vi "ReadAndProcessCommand.vi"(11 "MockGyroData In":T1={"BufferUpdateFIFO"="MockGyroBufferUpdate", "MockGyroCommandInput"="ModbusSubnetEGyroRxDataFIFO", "MockGyroDataOutput"="ModbusSubnetEGyroTxDataFIFO", "MockGyroDataRate"="MockGyroDataRateRegister", "MockGyroXValue"="MockGyroXValueRegister", "MockGyroYValue"="MockGyroYValueRegister", "MockGyroZValue"="MockGyroZValueRegister", "MockGyroStatus"="MockGyroStatusRegister", "MockGyroTemperature"="MockGyroTemperatureRegister", "CRCDataFIFO"="MockGyroCRCDataFIFO", "CRCCalculateFIFO"="MockGyroCRCCalculateFIFO", "CRCFIFO"="MockGyroCRCFIFO", "MockGyroCommandReplyFIFO"="MockGyroCommandReplyFIFO", "MockGyroReplyReadyFIFO"="MockGyroReplyReadyFIFO", "MockGyroModeFIFO"="MockGyroModeFIFO"}) -> ()   [LabVIEW 2016, in "FPGAMockGyro.lvlib"]
uses:
  FPGAMockGyro.lvlib
  DataTypes/MockGyroData.ctl
  DataTypes/MockGyroModes.ctl
  <vilib>/rvi/Emulation/niFpgaGetClockAttributes.vi
  <vilib>/rvi/Emulation/niFpgaSctlEmulationGetInTimedLoop.vi
  <vilib>/rvi/Emulation/niFpgaEmulationReportErrorSimple.vi
  <vilib>/rvi/DataTransferAndStorage/Container/Common/niFpgaContainerExecOnDevCompGetState.vi
  <vilib>/rvi/Emulation/niFpgaEmulationIsFPGAContextNoSignature.vi
  <vilib>/rvi/errors/niFpgaSetErrorForExecOnDevCompSimple.vi
  <vilib>/rvi/eio/common/nirviEmuReportErrorAndStop.vi
  <vilib>/rvi/DataTransferAndStorage/Container/Common/niFpgaContainerGetUniqueNameForEmu.vi
  <vilib>/rvi/FIFO/Fifo_Resource/nirvififoEmulationSetSize.vi
  <vilib>/rvi/FIFO/Fifo_Resource/nirviFifoEmulationQueueMgr.vi
  <instcachedir>/0/nirviFifoEmulationQueueMgr_E5CAEC123FF24DC58D834DCA3CDAA9B5.lvgen/nirviFifoEmulationQueueMgr_E5CAEC123FF24DC58D834DCA3CDAA9B5_002.vi
  <vilib>/rvi/FIFO/Fifo_Resource/nirvififoEmulationDetermineInputValidOut.vi
  <vilib>/rvi/FIFO/Fifo_Resource/nirvififoEmulationCreateLock.vi
  <vilib>/rvi/Emulation/niFpgaProcessEmulError.vi
  <vilib>/rvi/FIFO/Fifo_Resource/nirvififoEmulationObtainLock.vi
  <vilib>/rvi/FIFO/Fifo_Resource/nirvififoEmulationReleaseLock.vi
  <vilib>/rvi/occurrence/nirviWaitOnOccurrenceBase.vi
  <vilib>/rvi/errors/nirviReportUnexpectedCaseInternalError.vi
  <vilib>/rvi/errors/nirviReportUnexpectedCaseInternalError (U32).vi
  <vilib>/Utility/error.llb/Clear Errors.vi
  <vilib>/rvi/interface/RandomDataEmulation/niFpgaRandomDataHandleErrors.vi
  <instcachedir>/0/nirviFifoEmulationQueueMgr_E5CAEC123FF24DC58D834DCA3CDAA9B5.lvgen/nirviFifoEmulationQueueMgr_E5CAEC123FF24DC58D834DCA3CDAA9B5_000.vi
  <vilib>/rvi/Emulation/niFpgaCriticalErrorInLSC.vi
  <vilib>/rvi/Memory/Memory_Emulation/niFpgaMemoryEmulationCacheClearOnFirstRun.vi
  <vilib>/rvi/Memory/Memory_Emulation/nirvimemoryEmulationManagerCache_MakeExclusive.vi
  <vilib>/rvi/Memory/Memory_Emulation/niFpgaMemoryEmulationValidateCache.vi
  <vilib>/rvi/Memory/Memory_Emulation/nirvimemoryEmulationManagerCache_InsertValue.vi
  <vilib>/rvi/Memory/Memory_Emulation/nirvimemoryEmulationManagerCache_ReleaseExclusive.vi
  <vilib>/rvi/Memory/Memory_Emulation/nirvimemoryEmulationManagerCache_GetValue.vi
  <vilib>/rvi/Memory/Memory_Emulation/nirvimemoryEmulationManagerCache_SetValue.vi
  <instcachedir>/0/nirviFifoEmulationQueueMgr_E5CAEC123FF24DC58D834DCA3CDAA9B5.lvgen/nirviFifoEmulationQueueMgr_E5CAEC123FF24DC58D834DCA3CDAA9B5_001.vi
  <vilib>/rvi/DataTransferAndStorage/Container/XNode/niFpgaContainer.xnode
  <vilib>/rvi/FIFO/Fifo_Resource/niFpgaFifoEmulationRefIn.vi
  <vilib>/rvi/DataTransferAndStorage/Register/Emulation/niFpgaRegisterEmulationRefIn.vi
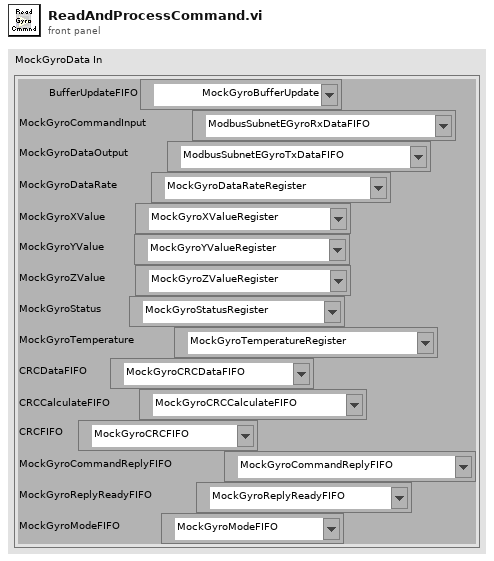
[diagram p1: front panel]
types:
  T1 = typedef "FPGAMockGyro.lvlib/MockGyroData.ctl" = cluster{"BufferUpdateFIFO":refnum<k21>, "MockGyroCommandInput":refnum<k21>, "MockGyroDataOutput":refnum<k21>, "MockGyroDataRate":refnum<k21>, "MockGyroXValue":refnum<k21>, "MockGyroYValue":refnum<k21>, "MockGyroZValue":refnum<k21>, "MockGyroStatus":refnum<k21>, "MockGyroTemperature":refnum<k21>, "CRCDataFIFO":refnum<k21>, "CRCCalculateFIFO":refnum<k21>, "CRCFIFO":refnum<k21>, "MockGyroCommandReplyFIFO":refnum<k21>, "MockGyroReplyReadyFIFO":refnum<k21>, "MockGyroModeFIFO":refnum<k21>}
  T2 = typedef "FPGAMockGyro.lvlib/MockGyroModes.ctl" = enum8{"Normal", "Config"}
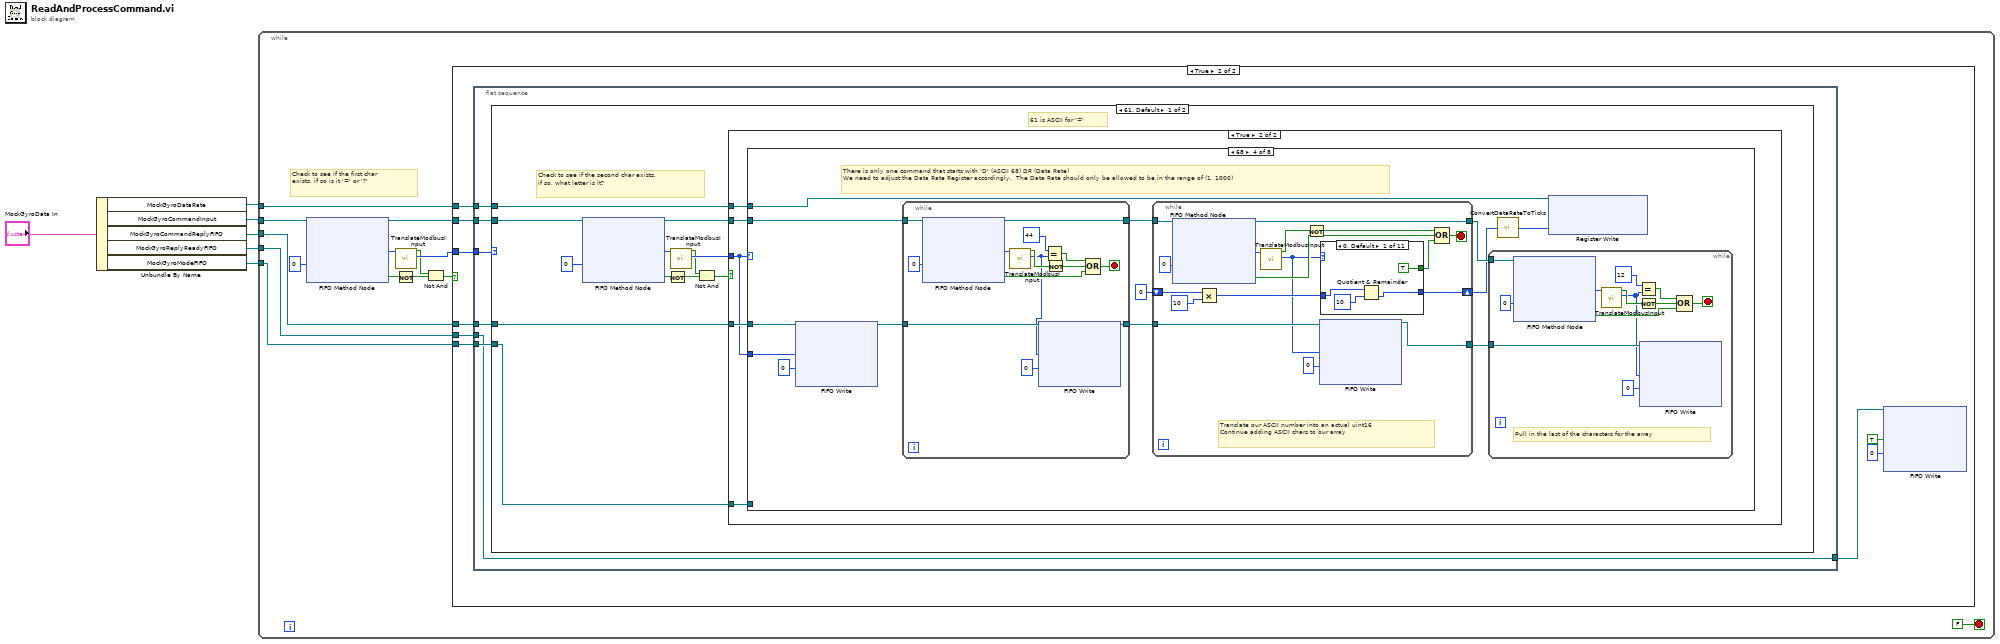
[diagram p0: block diagram]
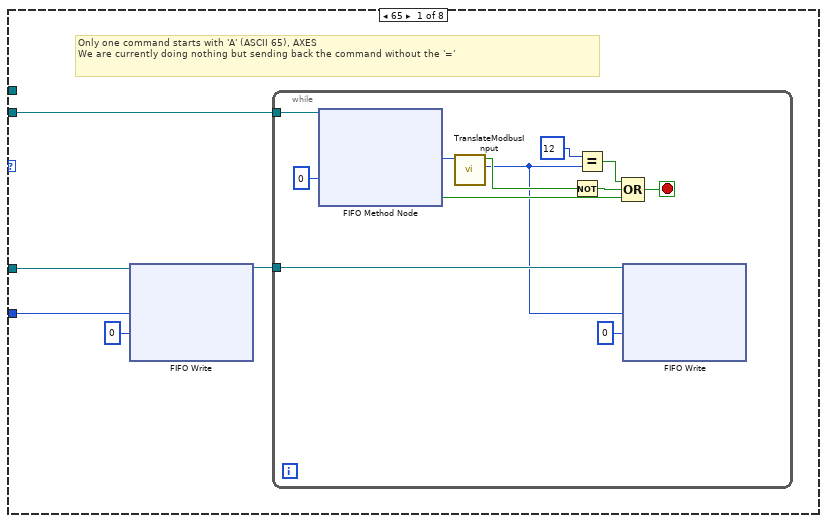
[diagram p4: hidden frame]
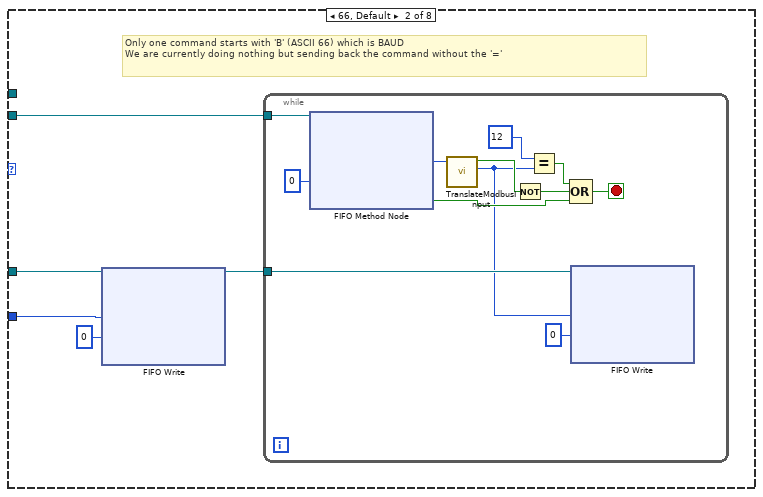
[diagram p5: hidden frame]
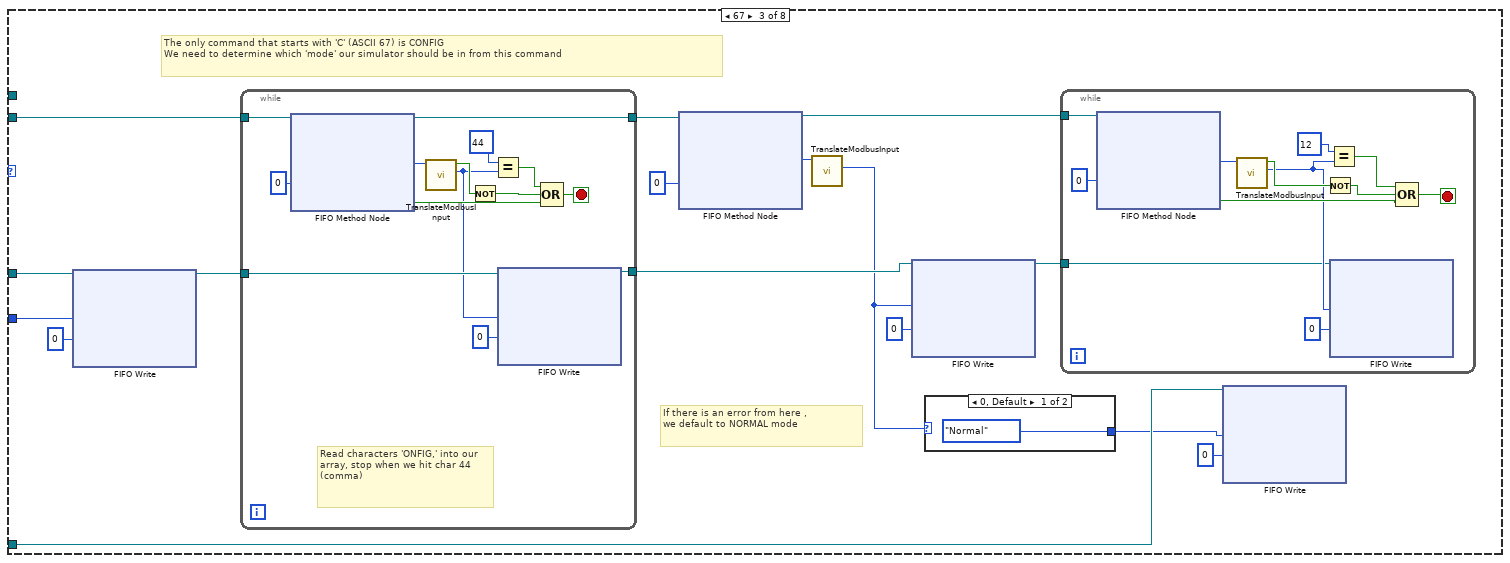
[diagram p6: hidden frame]
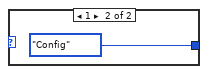
[diagram p7: hidden frame]
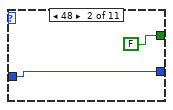
[diagram p8: hidden frame]
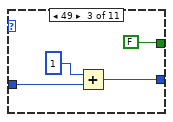
[diagram p9: hidden frame]
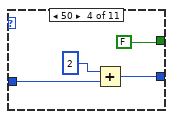
[diagram p10: hidden frame]
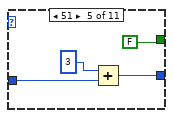
[diagram p11: hidden frame]
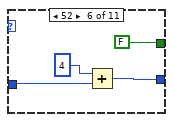
[diagram p12: hidden frame]
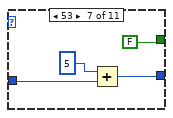
[diagram p13: hidden frame]
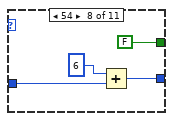
[diagram p14: hidden frame]
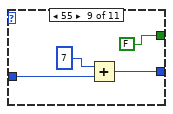
[diagram p15: hidden frame]
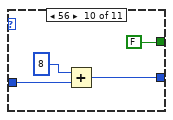
[diagram p16: hidden frame]
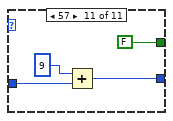
[diagram p17: hidden frame]
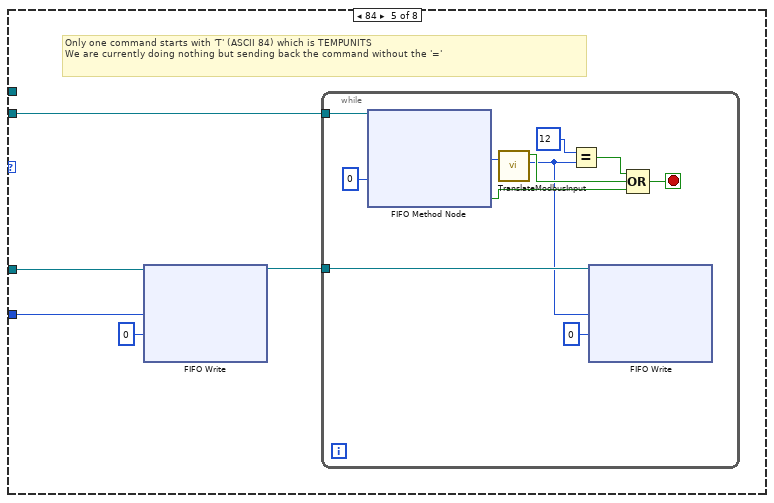
[diagram p18: hidden frame]
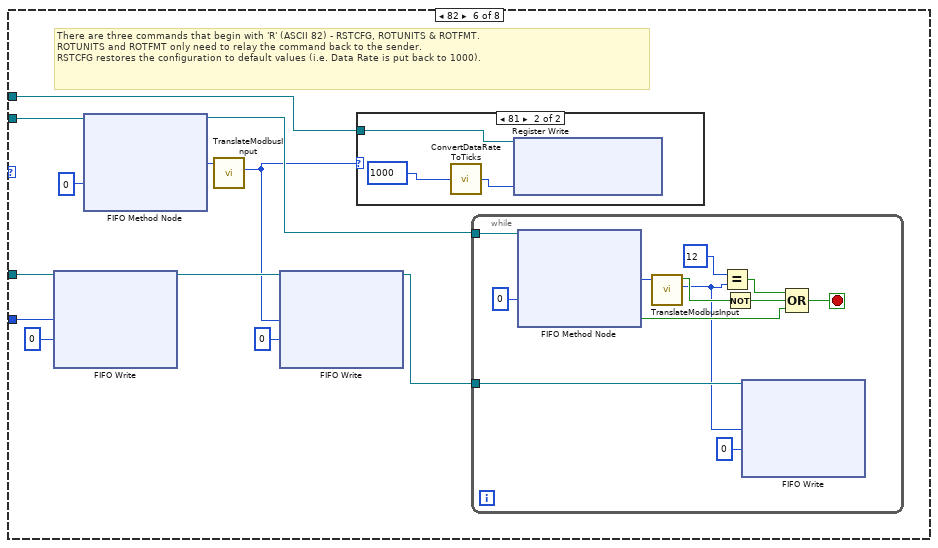
[diagram p19: hidden frame]
diagram:
  n1 = Unbundle By Name("MockGyroData In") -> ("MockGyroDataRate"=w4:refnum<k21>, "MockGyroCommandInput"=w6:refnum<k21>, "MockGyroCommandReplyFIFO"=w3:refnum<k21>, "MockGyroReplyReadyFIFO"=w2:refnum<k21>, "MockGyroModeFIFO"=w1:refnum<k21>)
  n2 = while {
    tunnel: w6 -> [w19]
    tunnel: w4 -> [w17]
    tunnel: w3 -> [w9]
    tunnel: w2 -> [w8]
    tunnel: w1 -> [w7]
    stop <- FALSE stop-if-true
    # "Check to see if the first char \nexists, if so is it '=' or '?'"
    n3 = xnode ("FIFO Method Node")("Timeout"=0, "FIFO In"=w19) -> ("Element"=w16:u16, "Timed Out?"=w14:bool, "FIFO Out"=w18:refnum<k21>)
    n4 = call "TranslateModbusInput.vi"("ModbusInput"=w16) -> ("ASCII Number Output"=w15:u8, "Is Data?"=w12:bool)  [unwired: 9 in]
    n5 = Not(x=w14) -> (.not. x?=w11:bool)
    n6 = Not And(1:w11, 2:w12) -> (0:w13:bool)
    n7 = case shown="True" w13 {
      tunnel: w18 -> [_ w29]
      tunnel: w17 -> [_ w28]
      tunnel: w15 -> [_ w27]
      tunnel: w9 -> [_ w26]
      tunnel: w8 -> [_ w23]
      tunnel: w7 -> [_ w25]
      frame False {
      }
      frame True {
        n8 = flat-sequence {
          tunnel: w29 -> [w35]
          tunnel: w28 -> [w34]
          tunnel: w27 -> [w33]
          tunnel: w26 -> [w32]
          tunnel: w25 -> [w31]
          tunnel: w23 -> [w30]
          tunnel: [w30] -> w22
          frame #0 {
            n9 = case shown="61, Default" w33 {
              tunnel: w35 -> [w47 w325]
              tunnel: w34 -> [w44 _]
              tunnel: w32 -> [w37 w324]
              tunnel: w31 -> [w36 _]
              frame 61, Default {
                # "Check to see if the second char exists,\nif so, what letter is it?"
                # "61 is ASCII for '='"
                n10 = xnode ("FIFO Method Node")("Timeout"=0, "FIFO In"=w47) -> ("Element"=w43:u16, "Timed Out?"=w40:bool, "FIFO Out"=w45:refnum<k21>)
                n11 = Not(x=w40) -> (.not. x?=w41:bool)
                n12 = call "TranslateModbusInput.vi"("ModbusInput"=w43) -> ("ASCII Number Output"=w42:u8, "Is Data?"=w39:bool)  [unwired: 9 in]
                n13 = Not And(1:w41, 2:w39) -> (0:w38:bool)
                n14 = case shown="True" w38 {
                  tunnel: w45 -> [_ w52]
                  tunnel: w44 -> [_ w51]
                  tunnel: w42 -> [_ w49]
                  tunnel: w37 -> [_ w50]
                  tunnel: w36 -> [_ w48]
                  frame False {
                  }
                  frame True {
                    n15 = case shown="68" w49 {
                      tunnel: w52 -> [w57 w74 w101 w143 w233 w256 w276 w293]
                      tunnel: w51 -> [_ _ _ w139 _ w253 _ _]
                      tunnel: w50 -> [w56 w73 w98 w138 w232 w251 w274 w292]
                      tunnel: w49 -> [w55 w72 w97 w137 w231 w249 w273 w291]
                      tunnel: w48 -> [_ _ w89 _ _ _ _ _]
                      frame 65 {
                        # "Only one command starts with 'A' (ASCII 65), AXES\nWe are currently doing nothing but sending back the command without the '='"
                        n16 = xnode ("FIFO Write")("Element"=w55, "Timeout"=0, "FIFO In"=w56) -> ("FIFO Out"=w53:refnum<k21>)  [unwired: 1 out]
                        n17 = while {
                          tunnel: w57 -> [w69]
                          tunnel: w53 -> [w60]
                          stop <- w61 stop-if-true
                          n18 = xnode ("FIFO Method Node")("Timeout"=0, "FIFO In"=w69) -> ("Element"=w67:u16, "Timed Out?"=w62:bool)  [unwired: 1 out]
                          n19 = call "TranslateModbusInput.vi"("ModbusInput"=w67) -> ("ASCII Number Output"=w59:u8, "Is Data?"=w64:bool)  [unwired: 9 in]
                          n20 = Not(x=w64) -> (.not. x?=w63:bool)
                          n21 = Equal?(x=u8 12, y=w59) -> (x = y?=w65:bool)
                          n22 = Compound Arithmetic op=OR(w65, w63, w62) -> (w61:bool)
                          n23 = xnode ("FIFO Write")("Element"=w59, "Timeout"=0, "FIFO In"=w60) -> ()  [unwired: 2 out]
                        }
                      }
                      frame 66, Default {
                        # "Only one command starts with 'B' (ASCII 66) which is BAUD\nWe are currently doing nothing but sending back the command without the '='"
                        n24 = xnode ("FIFO Write")("Element"=w72, "Timeout"=0, "FIFO In"=w73) -> ("FIFO Out"=w70:refnum<k21>)  [unwired: 1 out]
                        n25 = while {
                          tunnel: w74 -> [w86]
                          tunnel: w70 -> [w77]
                          stop <- w78 stop-if-true
                          n26 = xnode ("FIFO Method Node")("Timeout"=0, "FIFO In"=w86) -> ("Element"=w84:u16, "Timed Out?"=w79:bool)  [unwired: 1 out]
                          n27 = call "TranslateModbusInput.vi"("ModbusInput"=w84) -> ("ASCII Number Output"=w76:u8, "Is Data?"=w81:bool)  [unwired: 9 in]
                          n28 = Not(x=w81) -> (.not. x?=w80:bool)
                          n29 = Equal?(x=u8 12, y=w76) -> (x = y?=w82:bool)
                          n30 = Compound Arithmetic op=OR(w82, w80, w79) -> (w78:bool)
                          n31 = xnode ("FIFO Write")("Element"=w76, "Timeout"=0, "FIFO In"=w77) -> ()  [unwired: 2 out]
                        }
                      }
                      frame 67 {
                        # "If there is an error from here ,\nwe default to NORMAL mode"
                        # "The only command that starts with 'C' (ASCII 67) is CONFIG\nWe need to determine which 'mode' our simulator should be in from this command"
                        n32 = xnode ("FIFO Write")("Element"=w97, "Timeout"=0, "FIFO In"=w98) -> ("FIFO Out"=w95:refnum<k21>)  [unwired: 1 out]
                        n33 = while {
                          tunnel: w101 -> [w128]
                          tunnel: [w126] -> w99
                          tunnel: w95 -> [w118]
                          tunnel: [w115] -> w94
                          stop <- w119 stop-if-true
                          # "Read characters 'ONFIG,' into our array, stop when we hit char 44 (comma)"
                          n34 = xnode ("FIFO Method Node")("Timeout"=0, "FIFO In"=w128) -> ("Element"=w125:u16, "Timed Out?"=w120:bool, "FIFO Out"=w126:refnum<k21>)
                          n35 = call "TranslateModbusInput.vi"("ModbusInput"=w125) -> ("ASCII Number Output"=w117:u8, "Is Data?"=w122:bool)  [unwired: 9 in]
                          n36 = Not(x=w122) -> (.not. x?=w121:bool)
                          n37 = Equal?(x=u8 44, y=w117) -> (x = y?=w123:bool)
                          n38 = xnode ("FIFO Write")("Element"=w117, "Timeout"=0, "FIFO In"=w118) -> ("FIFO Out"=w115:refnum<k21>)  [unwired: 1 out]
                          n39 = Compound Arithmetic op=OR(w123, w121, w120) -> (w119:bool)
                        }
                        n40 = xnode ("FIFO Method Node")("Timeout"=0, "FIFO In"=w99) -> ("Element"=w100:u16, "FIFO Out"=w91:refnum<k21>)  [unwired: 1 out]
                        n41 = call "TranslateModbusInput.vi"("ModbusInput"=w100) -> ("ASCII Number Output"=w92:u8)  [unwired: 9 in, 1 out]
                        n42 = xnode ("FIFO Write")("Element"=w92, "Timeout"=0, "FIFO In"=w94) -> ("FIFO Out"=w90:refnum<k21>)  [unwired: 1 out]
                        n43 = case shown="0, Default" w92 {
                          tunnel: [MockGyroModes."Normal" ("MockGyroModes") MockGyroModes."Config" ("MockGyroModes")] -> w87
                          frame 0, Default {
                          }
                          frame 1 {
                          }
                        }
                        n44 = while {
                          tunnel: w91 -> [w114]
                          tunnel: w90 -> [w103]
                          stop <- w106 stop-if-true
                          n45 = xnode ("FIFO Method Node")("Timeout"=0, "FIFO In"=w114) -> ("Element"=w112:u16, "Timed Out?"=w110:bool)  [unwired: 1 out]
                          n46 = call "TranslateModbusInput.vi"("ModbusInput"=w112) -> ("ASCII Number Output"=w105:u8, "Is Data?"=w108:bool)  [unwired: 9 in]
                          n47 = Not(x=w108) -> (.not. x?=w107:bool)
                          n48 = Equal?(x=u16 12, y=w105) -> (x = y?=w111:bool)
                          n49 = xnode ("FIFO Write")("Element"=w105, "Timeout"=0, "FIFO In"=w103) -> ()  [unwired: 2 out]
                          n50 = Compound Arithmetic op=OR(w111, w107, w110) -> (w106:bool)
                        }
                        n51 = xnode ("FIFO Write")("Element"=w87, "Timeout"=0, "FIFO In"=w89) -> ()  [unwired: 2 out]
                      }
                      frame 68 {
                        # "There is only one command that starts with 'D' (ASCII 68) DR (Data Rate)\nWe need to adjust the Data Rate Register accordingly.  The Data Rate should only be allowed to be in the range of (1, 1000)"
                        n52 = xnode ("FIFO Write")("Element"=w137, "Timeout"=0, "FIFO In"=w138) -> ("FIFO Out"=w135:refnum<k21>)  [unwired: 1 out]
                        n53 = while {
                          tunnel: w143 -> [w228]
                          tunnel: [w226] -> w142
                          tunnel: w135 -> [w218]
                          tunnel: [w215] -> w134
                          stop <- w219 stop-if-true
                          n54 = xnode ("FIFO Method Node")("Timeout"=0, "FIFO In"=w228) -> ("Element"=w225:u16, "Timed Out?"=w220:bool, "FIFO Out"=w226:refnum<k21>)
                          n55 = call "TranslateModbusInput.vi"("ModbusInput"=w225) -> ("ASCII Number Output"=w217:u8, "Is Data?"=w222:bool)  [unwired: 9 in]
                          n56 = xnode ("FIFO Write")("Element"=w217, "Timeout"=0, "FIFO In"=w218) -> ("FIFO Out"=w215:refnum<k21>)  [unwired: 1 out]
                          n57 = Equal?(x=u8 44, y=w217) -> (x = y?=w223:bool)
                          n58 = Not(x=w222) -> (.not. x?=w221:bool)
                          n59 = Compound Arithmetic op=OR(w223, w221, w220) -> (w219:bool)
                        }
                        n60 = while {
                          tunnel: w142 -> [w170]
                          shift-right: [w166] -> w132
                          shift-left: u16 0 -> [w169]
                          tunnel: [w160] -> w140
                          tunnel: w134 -> [w159]
                          tunnel: [w156] -> w133
                          stop <- w165 stop-if-true
                          # "Translate our ASCII number into an actual uint16\nContinue adding ASCII chars to our array"
                          n61 = xnode ("FIFO Method Node")("Timeout"=0, "FIFO In"=w170) -> ("Element"=w172:u16, "Timed Out?"=w162:bool, "FIFO Out"=w160:refnum<k21>)
                          n62 = Multiply(x=w169, y=u16 10) -> (x*y=w167:u16)
                          n63 = call "TranslateModbusInput.vi"("ModbusInput"=w172) -> ("ASCII Number Output"=w157:u8, "Is Data?"=w164:bool)  [unwired: 9 in]
                          n64 = Not(x=w164) -> (.not. x?=w163:bool)
                          n65 = xnode ("FIFO Write")("Element"=w157, "Timeout"=0, "FIFO In"=w159) -> ("FIFO Out"=w156:refnum<k21>)  [unwired: 1 out]
                          n66 = case shown="0, Default" w157 {
                            tunnel: w167 -> [w176 w178 w182 w185 w190 w193 w197 w201 w205 w209 w213]
                            tunnel: [w174 w178 w180 w184 w188 w192 w196 w200 w204 w208 w212] -> w166
                            tunnel: [TRUE FALSE FALSE FALSE FALSE FALSE FALSE FALSE FALSE FALSE FALSE] -> w161
                            frame 0, Default {
                              n67 = Quotient & Remainder(x=w176, y=u16 10) -> (floor(x/y)=w174:u16)  [unwired: 1 out]
                            }
                            frame 48 {
                            }
                            frame 49 {
                              n68 = Add(x=u16 1, y=w182) -> (x+y=w180:u16)
                            }
                            frame 50 {
                              n69 = Add(x=u16 2, y=w185) -> (x+y=w184:u16)
                            }
                            frame 51 {
                              n70 = Add(x=u16 3, y=w190) -> (x+y=w188:u16)
                            }
                            frame 52 {
                              n71 = Add(x=u16 4, y=w193) -> (x+y=w192:u16)
                            }
                            frame 53 {
                              n72 = Add(x=u16 5, y=w197) -> (x+y=w196:u16)
                            }
                            frame 54 {
                              n73 = Add(x=u16 6, y=w201) -> (x+y=w200:u16)
                            }
                            frame 55 {
                              n74 = Add(x=u16 7, y=w205) -> (x+y=w204:u16)
                            }
                            frame 56 {
                              n75 = Add(x=u16 8, y=w209) -> (x+y=w208:u16)
                            }
                            frame 57 {
                              n76 = Add(x=u16 9, y=w213) -> (x+y=w212:u16)
                            }
                          }
                          n77 = Compound Arithmetic op=OR(w163, w162, w161) -> (w165:bool)
                        }
                        n78 = while {
                          tunnel: w140 -> [w153]
                          tunnel: w133 -> [w146]
                          stop <- w152 stop-if-true
                          # "Pull in the last of the characters for the array"
                          n79 = xnode ("FIFO Method Node")("Timeout"=0, "FIFO In"=w153) -> ("Element"=w154:u16, "Timed Out?"=w147:bool)  [unwired: 1 out]
                          n80 = call "TranslateModbusInput.vi"("ModbusInput"=w154) -> ("ASCII Number Output"=w145:u8, "Is Data?"=w149:bool)  [unwired: 9 in]
                          n81 = Equal?(x=u8 12, y=w145) -> (x = y?=w150:bool)
                          n82 = Not(x=w149) -> (.not. x?=w148:bool)
                          n83 = xnode ("FIFO Write")("Element"=w145, "Timeout"=0, "FIFO In"=w146) -> ()  [unwired: 2 out]
                          n84 = Compound Arithmetic op=OR(w150, w148, w147) -> (w152:bool)
                        }
                        n85 = call "ConvertDataRateToTicks.vi"("DataRate"=w132) -> ("Ticks"=w131:u64)
                        n86 = xnode ("Register Write")("Data"=w131, "Register In"=w139) -> ()  [unwired: 1 out]
                      }
                      frame 84 {
                        # "Only one command starts with 'T' (ASCII 84) which is TEMPUNITS\nWe are currently doing nothing but sending back the command without the '='"
                        n87 = xnode ("FIFO Write")("Element"=w231, "Timeout"=0, "FIFO In"=w232) -> ("FIFO Out"=w229:refnum<k21>)  [unwired: 1 out]
                        n88 = while {
                          tunnel: w233 -> [w244]
                          tunnel: w229 -> [w236]
                          stop <- w237 stop-if-true
                          n89 = xnode ("FIFO Method Node")("Timeout"=0, "FIFO In"=w244) -> ("Element"=w242:u16, "Timed Out?"=w238:bool)  [unwired: 1 out]
                          n90 = call "TranslateModbusInput.vi"("ModbusInput"=w242) -> ("ASCII Number Output"=w234:u8, "Is Data?"=w239:bool)  [unwired: 9 in]
                          n91 = Equal?(x=u8 12, y=w234) -> (x = y?=w240:bool)
                          n92 = xnode ("FIFO Write")("Element"=w234, "Timeout"=0, "FIFO In"=w236) -> ()  [unwired: 2 out]
                          n93 = Compound Arithmetic op=OR(w240, w239, w238) -> (w237:bool)
                        }
                      }
                      frame 82 {
                        # "There are three commands that begin with 'R' (ASCII 82) - RSTCFG, ROTUNITS & ROTFMT.\nROTUNITS and ROTFMT only need to relay the command back to the sender.\nRSTCFG restores the configuration to default values (i.e. Data Rate is put back to 1000)."
                        n94 = xnode ("FIFO Write")("Element"=w249, "Timeout"=0, "FIFO In"=w251) -> ("FIFO Out"=w248:refnum<k21>)  [unwired: 1 out]
                        n95 = xnode ("FIFO Method Node")("Timeout"=0, "FIFO In"=w256) -> ("Element"=w252:u16, "FIFO Out"=w254:refnum<k21>)  [unwired: 1 out]
                        n96 = call "TranslateModbusInput.vi"("ModbusInput"=w252) -> ("ASCII Number Output"=w247:u8)  [unwired: 9 in, 1 out]
                        n97 = xnode ("FIFO Write")("Element"=w247, "Timeout"=0, "FIFO In"=w248) -> ("FIFO Out"=w245:refnum<k21>)  [unwired: 1 out]
                        n98 = case shown="81" w247 {
                          tunnel: w253 -> [_ w271]
                          frame 79, Default {
                          }
                          frame 81 {
                            n99 = call "ConvertDataRateToTicks.vi"("DataRate"=u16 1000 ("Data")) -> ("Ticks"=w269:u64)
                            n100 = xnode ("Register Write")("Data"=w269, "Register In"=w271) -> ()  [unwired: 1 out]
                          }
                        }
                        n101 = while {
                          tunnel: w254 -> [w268]
                          tunnel: w245 -> [w259]
                          stop <- w260 stop-if-true
                          n102 = xnode ("FIFO Method Node")("Timeout"=0, "FIFO In"=w268) -> ("Element"=w266:u16, "Timed Out?"=w261:bool)  [unwired: 1 out]
                          n103 = call "TranslateModbusInput.vi"("ModbusInput"=w266) -> ("ASCII Number Output"=w257:u8, "Is Data?"=w263:bool)  [unwired: 9 in]
                          n104 = Equal?(x=u8 12, y=w257) -> (x = y?=w264:bool)
                          n105 = Not(x=w263) -> (.not. x?=w262:bool)
                          n106 = xnode ("FIFO Write")("Element"=w257, "Timeout"=0, "FIFO In"=w259) -> ()  [unwired: 2 out]
                          n107 = Compound Arithmetic op=OR(w264, w262, w261) -> (w260:bool)
                        }
                      }
                      frame 70 {
                        # "There are three commands that begin with 'F' (ASCII 70) - FILTEN, FILTTYPE & FC.\nWe are only required to echo the command back to the sender."
                        n108 = xnode ("FIFO Write")("Element"=w273, "Timeout"=0, "FIFO In"=w274) -> ("FIFO Out"=w272:refnum<k21>)  [unwired: 1 out]
                        n109 = while {
                          tunnel: w276 -> [w288]
                          tunnel: w272 -> [w278]
                          stop <- w280 stop-if-true
                          n110 = xnode ("FIFO Method Node")("Timeout"=0, "FIFO In"=w288) -> ("Element"=w286:u16, "Timed Out?"=w281:bool)  [unwired: 1 out]
                          n111 = call "TranslateModbusInput.vi"("ModbusInput"=w286) -> ("ASCII Number Output"=w279:u8, "Is Data?"=w282:bool)  [unwired: 9 in]
                          n112 = xnode ("FIFO Write")("Element"=w279, "Timeout"=0, "FIFO In"=w278) -> ()  [unwired: 2 out]
                          n113 = Not(x=w282) -> (.not. x?=w283:bool)
                          n114 = Equal?(x=u8 12, y=w279) -> (x = y?=w284:bool)
                          n115 = Compound Arithmetic op=OR(w284, w283, w281) -> (w280:bool)
                        }
                      }
                      frame 77 {
                        # "Only one command starts with 'M' (ASCII 77) which is MSYNC\nWe are currently doing nothing but sending back the command without the '='"
                        n116 = xnode ("FIFO Write")("Element"=w291, "Timeout"=0, "FIFO In"=w292) -> ("FIFO Out"=w289:refnum<k21>)  [unwired: 1 out]
                        n117 = while {
                          tunnel: w293 -> [w305]
                          tunnel: w289 -> [w296]
                          stop <- w297 stop-if-true
                          n118 = xnode ("FIFO Method Node")("Timeout"=0, "FIFO In"=w305) -> ("Element"=w303:u16, "Timed Out?"=w298:bool)  [unwired: 1 out]
                          n119 = call "TranslateModbusInput.vi"("ModbusInput"=w303) -> ("ASCII Number Output"=w294:u8, "Is Data?"=w300:bool)  [unwired: 9 in]
                          n120 = Not(x=w300) -> (.not. x?=w299:bool)
                          n121 = Equal?(x=u8 12, y=w294) -> (x = y?=w302:bool)
                          n122 = xnode ("FIFO Write")("Element"=w294, "Timeout"=0, "FIFO In"=w296) -> ()  [unwired: 2 out]
                          n123 = Compound Arithmetic op=OR(w302, w299, w298) -> (w297:bool)
                        }
                      }
                    }
                  }
                }
              }
              frame 63 {
                # "\\n"
                # "2 or \\r"
                # "Since BIT (Built In Test) is the only one that starts with '?'\nWe don't need to worry about the other commands.\nWe will do the BIT processing here."
                # "63 is ASCII for '?'"
                n124 = while {
                  tunnel: w325 -> [w376]
                  tunnel: [w366] -> w322
                  stop <- w367 stop-if-true
                  # "Pull in the BIT, part from the input"
                  n125 = xnode ("FIFO Method Node")("Timeout"=0, "FIFO In"=w376) -> ("Element"=w374:u16, "Timed Out?"=w368:bool, "FIFO Out"=w366:refnum<k21>)
                  n126 = call "TranslateModbusInput.vi"("ModbusInput"=w374) -> ("ASCII Number Output"=w373:u8, "Is Data?"=w370:bool)  [unwired: 9 in]
                  n127 = Not(x=w370) -> (.not. x?=w369:bool)
                  n128 = Equal?(x=u8 44, y=w373) -> (x = y?=w372:bool)
                  n129 = Compound Arithmetic op=OR(w372, w369, w368) -> (w367:bool)
                }
                n130 = for {
                  tunnel: w324 -> [w365]
                  tunnel: u8[] [254, 129, 0] -> [w360] mode=indexing
                  tunnel: [w363] -> w308
                  shift-right: [w359] -> w316
                  shift-left: i16 0 -> [w362]
                  # "The HEADER always starts FE8100"
                  n131 = To Word Integer(number=w360) -> (16bit integer=w361:i16)
                  n132 = xnode ("FIFO Write")("Element"=w360, "Timeout"=0, "FIFO In"=w365) -> ("FIFO Out"=w363:refnum<k21>)  [unwired: 1 out]
                  n133 = Add(x=w361, y=w362) -> (x+y=w359:i16)
                }
                n134 = xnode ("FIFO Method Node")("Timeout"=0, "FIFO In"=w322) -> ("Element"=w319:u16, "FIFO Out"=w309:refnum<k21>)  [unwired: 1 out]
                n135 = case shown="32" w319 {
                  tunnel: w308 -> [w350 w357]
                  tunnel: w309 -> [_ w355]
                  tunnel: w316 -> [w347 w353]
                  tunnel: [w345 w351] -> w315
                  frame 0, Default {
                    w346 = u8 170 ("Element")
                    # "HEADER 'AA'"
                    n136 = To Word Integer(number=w346) -> (16bit integer=w348:i16)
                    n137 = xnode ("FIFO Write")("Element"=w346, "Timeout"=0, "FIFO In"=w350) -> ()  [unwired: 2 out]
                    n138 = Add(x=w348, y=w347) -> (x+y=w345:i16)
                  }
                  frame 32 {
                    w352 = u8 171 ("Element")
                    # "\\r"
                    # "HEADER 'AB'"
                    n139 = To Word Integer(number=w352) -> (16bit integer=w354:i16)
                    n140 = xnode ("FIFO Method Node")("Timeout"=0, "FIFO In"=w355) -> ()  [unwired: 3 out]
                    n141 = xnode ("FIFO Write")("Element"=w352, "Timeout"=0, "FIFO In"=w357) -> ()  [unwired: 2 out]
                    n142 = Add(x=w354, y=w353) -> (x+y=w351:i16)
                  }
                }
                n143 = xnode ("FIFO Method Node")("Timeout"=0, "FIFO In"=w309) -> ()  [unwired: 3 out]
                n144 = for {
                  tunnel: u8[] [127, 127, 127, 127, 127, 127] -> [w329] mode=indexing
                  tunnel: [w332] -> w307
                  shift-right: [w328] -> w314
                  shift-left: w315 -> [w330]
                  tunnel: w308 -> [w327]
                  # "7F7F7F7F7F7F"
                  n145 = To Word Integer(number=w329) -> (16bit integer=w331:i16)
                  n146 = xnode ("FIFO Write")("Element"=w329, "Timeout"=0, "FIFO In"=w327) -> ("FIFO Out"=w332:refnum<k21>)  [unwired: 1 out]
                  n147 = Add(x=w331, y=w330) -> (x+y=w328:i16)
                }
                n148 = case shown="32" w319 {
                  tunnel: w307 -> [_ w337]
                  tunnel: w314 -> [w333 w335]
                  tunnel: [w333 w334] -> w313
                  frame 0, Default {
                  }
                  frame 32 {
                    n149 = for {
                      tunnel: w337 -> [w343]
                      tunnel: u8[] [127, 127] -> [w341] mode=indexing
                      shift-right: [w339] -> w334
                      shift-left: w335 -> [w340]
                      tunnel: [w338] -> _
                      # "7F7F"
                      n150 = To Word Integer(number=w341) -> (16bit integer=w342:i16)
                      n151 = xnode ("FIFO Write")("Element"=w341, "Timeout"=0, "FIFO In"=w343) -> ("FIFO Out"=w338:refnum<k21>)  [unwired: 1 out]
                      n152 = Add(x=w342, y=w340) -> (x+y=w339:i16)
                    }
                  }
                }
                n153 = Quotient & Remainder(x=w313, y=i16 256) -> (x-y*floor(x/y)=w310:i16)  [unwired: 1 out]
                n154 = To Unsigned Byte Integer(number=w310) -> (unsigned 8bit integer=w311:u8)
                n155 = xnode ("FIFO Write")("Element"=w311, "Timeout"=0, "FIFO In"=w307) -> ()  [unwired: 2 out]
              }
            }
          }
        }
        n156 = xnode ("FIFO Write")("Element"=TRUE, "Timeout"=0, "FIFO In"=w22) -> ()  [unwired: 2 out]
      }
    }
  }
